vi "SW_Gen_Check_segments_parameters.vi"(3 "Image plotting parameters":T1) -> (1 "Corrected image plotting parameters":T1)   [LabVIEW 2016]
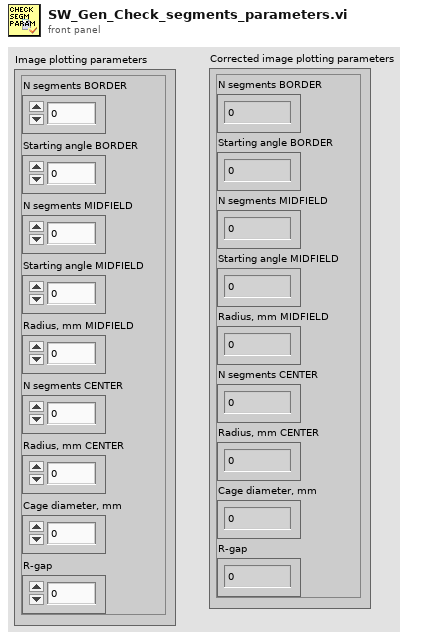
[diagram p1: front panel]
types:
  T1 = cluster{"N segments BORDER":u8, "Starting angle BORDER":i16, "N segments MIDFIELD":u8, "Starting angle MIDFIELD":i16, "Radius, mm MIDFIELD":u16, "N segments CENTER":u8, "Radius, mm CENTER":u16, "Cage diameter, mm":u16, "R-gap":i32}
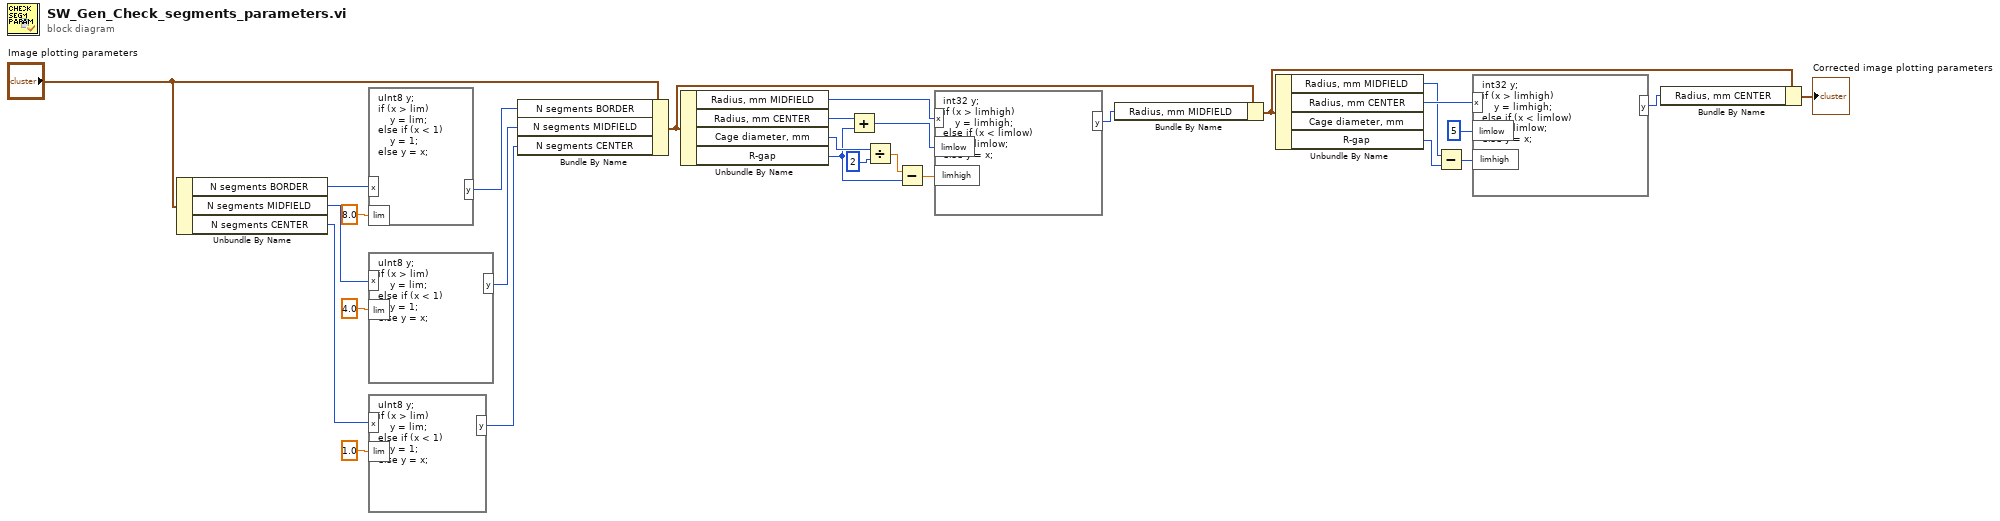
[diagram p0: block diagram]
diagram:
  n1 = Unbundle By Name("Image plotting parameters") -> ("N segments BORDER"=w28:u8, "N segments MIDFIELD"=w27:u8, "N segments CENTER"=w26:u8)
  n2 = formula code="uInt8 y;\nif (x > lim)\n    y = lim;\nelse if (x < 1)\n    y = 1;\nelse y = x;"("x"=w28, "lim"=8.0 ("input variable")) -> ("y"=w22:u8)
  n3 = formula code="uInt8 y;\nif (x > lim)\n    y = lim;\nelse if (x < 1)\n    y = 1;\nelse y = x;"("x"=w27, "lim"=4.0 ("input variable")) -> ("y"=w21:u8)
  n4 = formula code="uInt8 y;\nif (x > lim)\n    y = lim;\nelse if (x < 1)\n    y = 1;\nelse y = x;"("x"=w26, "lim"=1.0 ("input variable")) -> ("y"=w20:u8)
  n5 = Bundle By Name(cluster="Image plotting parameters", "N segments BORDER"=w22, "N segments MIDFIELD"=w21, "N segments CENTER"=w20) -> (w1:T1)
  n6 = Unbundle By Name(w1) -> ("Radius, mm MIDFIELD"=w19:u16, "Radius, mm CENTER"=w14:u16, "Cage diameter, mm"=w18:u16, "R-gap"=w13:i32)
  n7 = Add(x=w14, y=w13) -> (x+y=w12:i32)
  n8 = Divide(x=w18, y=u16 2) -> (x/y=w16:dbl)
  n9 = Subtract(x=w16, y=w13) -> (x-y=w15:dbl)
  n10 = formula code="int32 y;\nif (x > limhigh)\n    y = limhigh;\nelse if (x < limlow)\n    y = limlow;\nelse y = x;"("x"=w19, "limlow"=w12, "limhigh"=w15) -> ("y"=w11:i32)
  n11 = Bundle By Name(cluster=w1, "Radius, mm MIDFIELD"=w11) -> (w5:T1)
  n12 = Unbundle By Name(w5) -> ("Radius, mm MIDFIELD"=w8:u16, "Radius, mm CENTER"=w10:u16, "R-gap"=w7:i32)  [unwired: 1 out]
  n13 = Subtract(x=w8, y=w7) -> (x-y=w6:i32)
  n14 = formula code="int32 y;\nif (x > limhigh)\n    y = limhigh;\nelse if (x < limlow)\n    y = limlow;\nelse y = x;"("x"=w10, "limlow"=5 ("input variable"), "limhigh"=w6) -> ("y"=w4:i32)
  n15 = Bundle By Name(cluster=w5, "Radius, mm CENTER"=w4) -> (→"Corrected image plotting parameters":T1)
